vi "Teleop.vi"(10 "Match Info":T1={"Autonomous Elapsed Seconds"=0.0, "TeleOp Elapsed Seconds"=0.0, "Disabled Elapsed Seconds"=0.0, "Visited Autonomous"=FALSE, "Visited TeleOp"=FALSE, "Visited Disabled"=FALSE, "Autonomous Settings"={"Autonomous Style"=enum."Independent", "VI Refnum"=refnum}}, 11 "Call Context":T2) -> ()   [LabVIEW 2013]
doc: "This VI is called for each TeleOp packet received from the DS where the robot is not disabled. It is often used to read from the joysticks and update I/O or to update setpoints for timed control loops. It should complete and return within 20 milliseconds or it may miss DS packets."
uses:
  <vilib>/Rock Robotics/WPI/DriverStation/WPI_DriverStationDerivedRobotMode.ctl
  <vilib>/Rock Robotics/WPI/DriverStation/WPI_DriverStationMatch Info.ctl
  <vilib>/Rock Robotics/WPI/Solenoid/WPI_SolenoidValue.ctl
  <vilib>/Rock Robotics/WPI/Relay/WPI_RelayValue.ctl
  Robot Global Data.vi
  <vilib>/Rock Robotics/WPI/Joystick/WPI_JoystickGetSetRefNum.vi
  <vilib>/Rock Robotics/WPI/RobotDrive/WPI_RobotDriveGetSetRefNum.vi
  <vilib>/Rock Robotics/WPI/RobotDrive/WPI_RobotDriveArcadeDrive_Standard(NoSaturation).vi
  <vilib>/Rock Robotics/WPI/Solenoid/WPI_SolenoidSetEnum.vi
panel:
  out "Numeric 1":dbl(slide) scale=0.0..100.0
  out "Boolean 2":bool
  out "Boolean 1":bool
  # "display DB vars here"
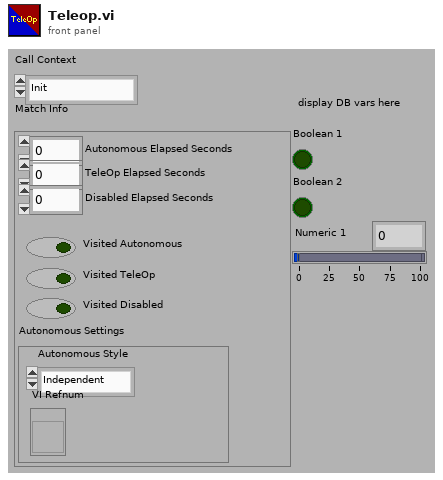
[diagram p1: front panel]
types:
  T1 = typedef "WPI_DriverStationMatch Info.ctl" = cluster{"Autonomous Elapsed Seconds":dbl, "TeleOp Elapsed Seconds":dbl, "Disabled Elapsed Seconds":dbl, "Visited Autonomous":bool, "Visited TeleOp":bool, "Visited Disabled":bool, "Autonomous Settings":cluster{"Autonomous Style":enum16{"Iterative", "Independent"}, "VI Refnum":refnum<vi>}}
  T2 = typedef "WPI_DriverStationDerivedRobotMode.ctl" = enum16{"Init", "Execute", "Stop"}
  T3 = typedef "WPI_JoystickDevRef.ctl" = cluster{"Device":T4}
  T4 = typedef "WPI_JoystickDeviceEnum.ctl" = enum16{"USB 1", "USB 2", "USB 3", "USB 4", "Kinect 1", "Kinect 2"}
  T5 = cluster{"axis 1 (x)":dbl, "axis 2 (y)":dbl, "axis 3 (throttle)":dbl, "axis 4":dbl, "axis 5":dbl, "axis 6":dbl}
  T6 = typedef "WPI_JoystickButtonState.ctl" = cluster{"Button 1":bool, "Button 2":bool, "Button 3":bool, "Button 4":bool, "Button 5":bool, "Button 6":bool, "Button 7":bool, "Button 8":bool, "Button 9":bool, "Button 10":bool, "Button 11":bool, "Button 12":bool}
  T7 = typedef "WPI_PWMDeviceRef.ctl" = cluster{"DeviceStatus":errorcluster, "Digital Module":T8, "PWM Channel":T9}
  T8 = typedef "FPGA_TypedefDigitalModule.ctl" = enum16{"Digital Module 1", "Digital Module 2"}
  T9 = typedef "FPGA_DIOPWMChannel.ctl" = enum8{"PWM 1", "PWM 2", "PWM 3", "PWM 4", "PWM 5", "PWM 6", "PWM 7", "PWM 8", "PWM 9", "PWM 10", "Invalid"}
  T10 = typedef "WPI_DigitalOutputDevRef.ctl" = cluster{"Digital Module":T8, "DIO Channel":T11, "DevStatus":errorcluster}
  T11 = typedef "FPGA_DIOChannel.ctl" = enum8{"DIO 1", "DIO 2", "DIO 3", "DIO 4", "DIO 5", "DIO 6", "DIO 7", "DIO 8", "DIO 9", "DIO 10", "DIO 11", "DIO 12", "DIO 13", "DIO 14", "Invalid"}
  T12 = typedef "WPI_RobotDriveDevRef.ctl" = cluster{"DevStatus":errorcluster, "Motors[]":T13[], "Square Inputs":bool, "Max Output":dbl, "Isochronous":bool}
  T13 = typedef "WPI_MotorControlDeviceRef.ctl" = cluster{"DeviceStatus":errorcluster, "Type":enum16{"PWM", "CAN"}, "PWM":cluster{"Digital Module":T8, "PWM Channel":T9, "DeadBand":T14}, "CAN":cluster{"Device Number":u8, "Control Mode":T15, "Semaphore":T16, "Max Vout":dbl}, "Invert":bool, "TransformRef":T17, "InvTransformRef":T17}
  T14 = typedef "WPI_PWMDeadband.ctl" = cluster{"Name":string, "maxPositivePwm":i32, "minPositivePwm":i32, "centerPwm":i32, "maxNegativePwm":i32, "minNegativePwm":i32, "angularRange":u16}
  T15 = typedef "WPI_CANJaguar_ControlMode.ctl" = enum8{"Percent VBus", "Current", "Speed", "Position", "Voltage"}
  T16 = typedef "Semaphore RefNum" = refnum<k1>
  T17 = typedef "WPI_PWMTransform_ConPane.ctl" = refnum<vi>
  T18 = typedef "WPI_SolenoidValue.ctl" = enum16{"Off", "On", "Forward", "Reverse"}
  T19 = typedef "WPI_RelayValue.ctl" = enum16{"Off", "On", "Forward", "Reverse"}
  T20 = typedef "WPI_RelayDevRef.ctl" = cluster{"DevStatus":errorcluster, "Relay Channel":T21, "Digital Module":T8, "Relay Direction":T22}
  T21 = typedef "FPGA_DIORelayChannel.ctl" = enum8{"Relay 1", "Relay 2", "Relay 3", "Relay 4", "Relay 5", "Relay 6", "Relay 7", "Relay 8", "Invalid"}
  T22 = typedef "WPI_RelayDirection.ctl" = enum16{"Both directions", "Forward only", "Reverse only"}
  T23 = typedef "WPI_SolenoidDevRef.ctl" = cluster{"DevStatus":errorcluster, "Solenoid Module":T24, "Forward Solenoid Channel":T25, "Reverse Solenoid Channel":T25}
  T24 = typedef "FPGA_TypedefSolenoidModule.ctl" = enum16{"Solenoid Module 1", "Solenoid Module 2"}
  T25 = typedef "WPI_SolenoidChannel.ctl" = enum8{"Solenoid 1", "Solenoid 2", "Solenoid 3", "Solenoid 4", "Solenoid 5", "Solenoid 6", "Solenoid 7", "Solenoid 8", "Invalid"}
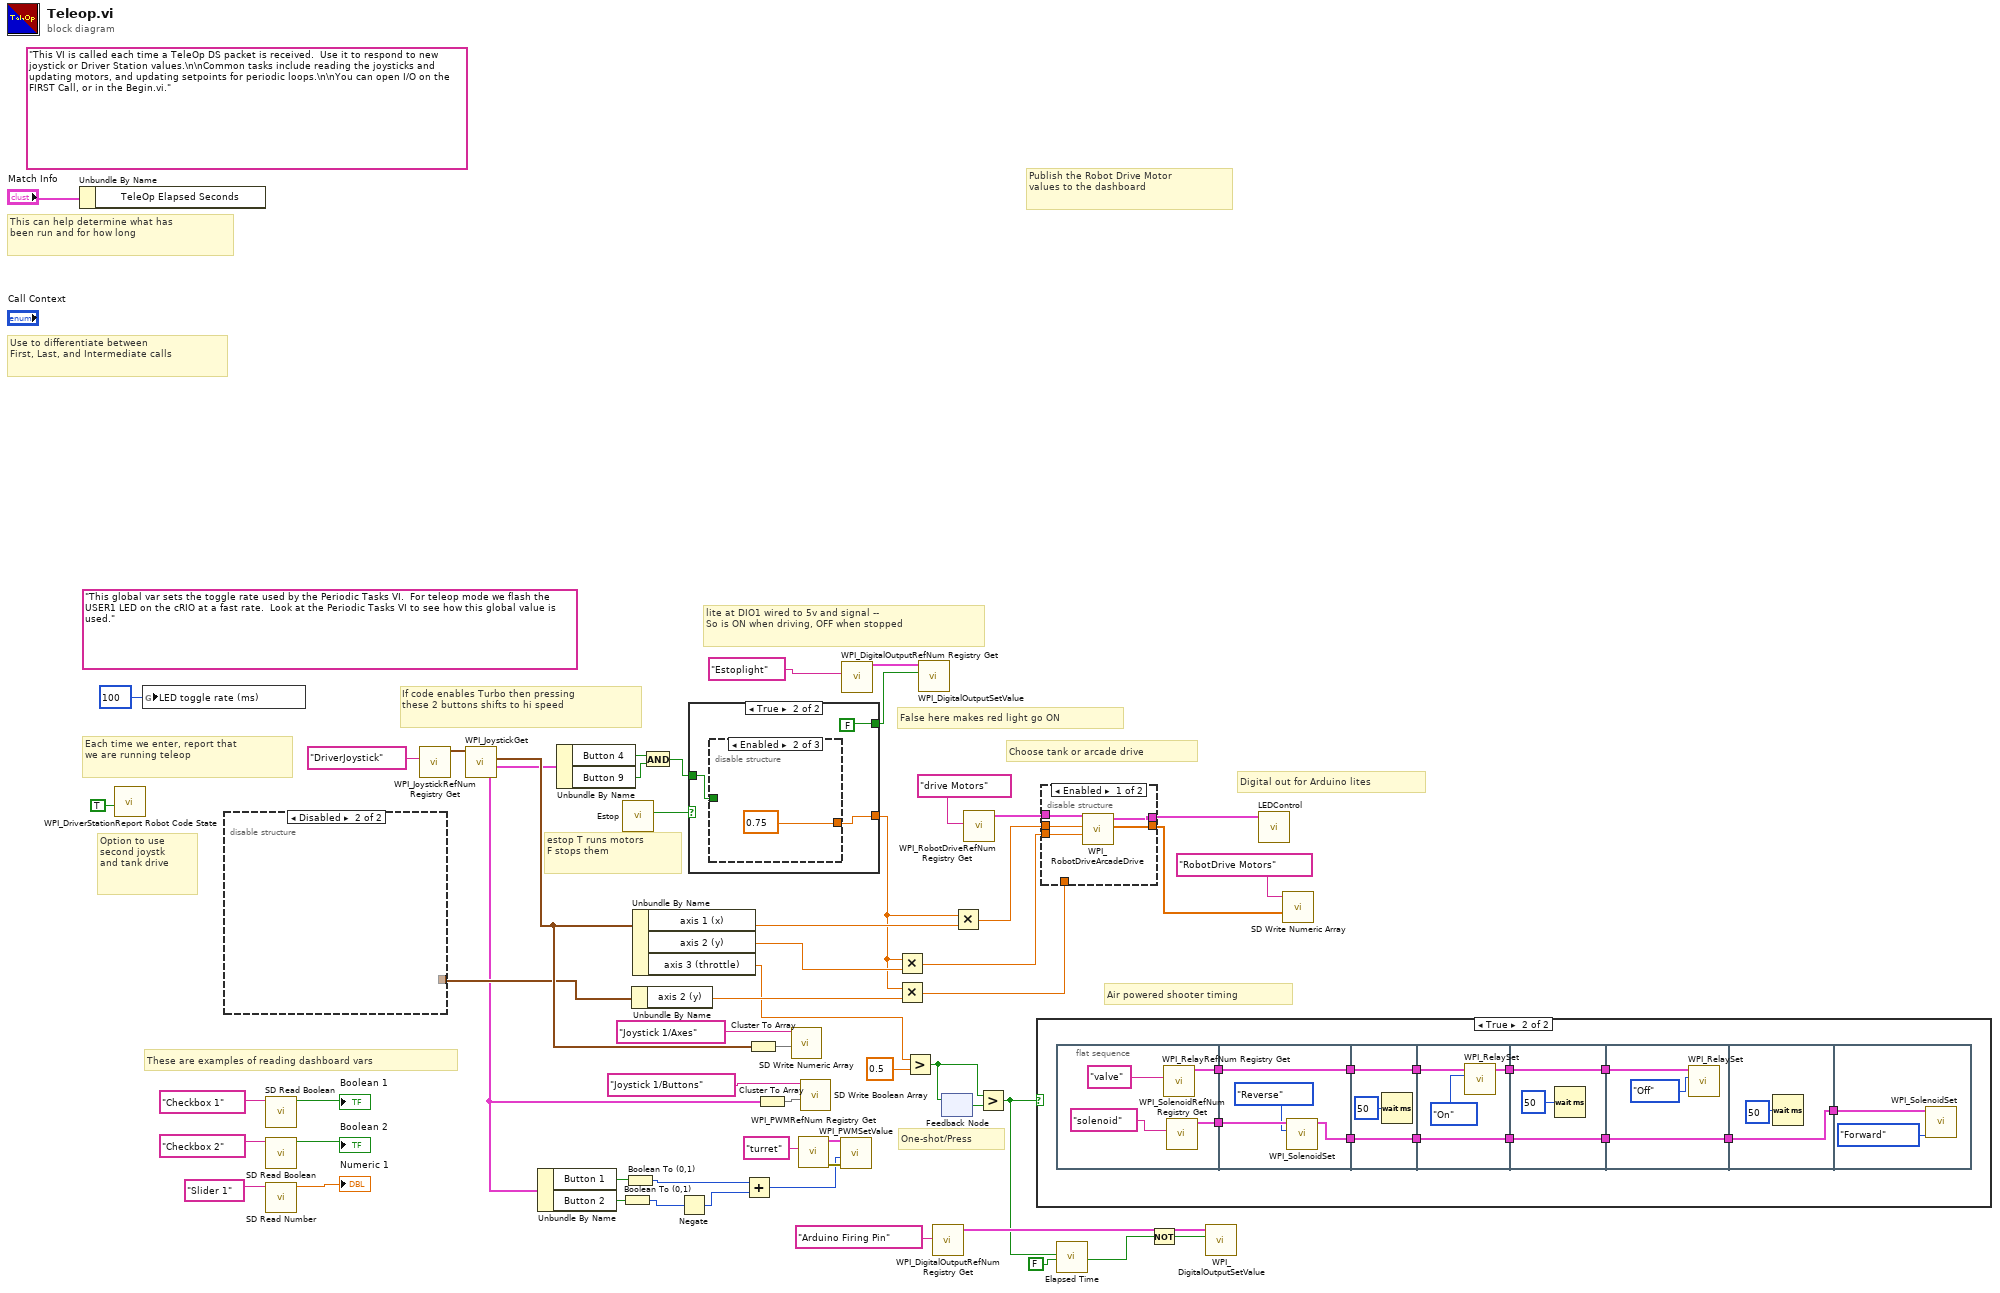
[diagram p0: block diagram]
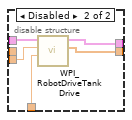
[diagram p3: hidden frame]
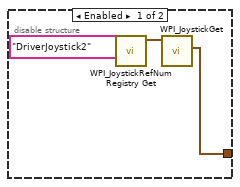
[diagram p4: hidden frame]
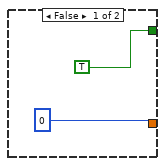
[diagram p5: hidden frame]
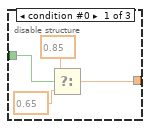
[diagram p6: hidden frame]
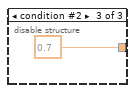
[diagram p7: hidden frame]
diagram:
  (unwired) "This global var sets the toggle rate used by the Periodic Tasks VI.  For teleop mode we flash the USER1 LED on the cRIO at a fast rate.  Look at the Periodic Tasks VI to see how this global value is used."
  (unwired) "This VI is called each time a TeleOp DS packet is received.  Use it to respond to new joystick or Driver Station values.\n\nCommon tasks include reading the joysticks and updating motors, and updating setpoints for periodic loops.\n\nYou can open I/O on the FIRST Call, or in the Begin.vi."
  # "Air powered shooter timing"
  # "False here makes red light go ON"
  # "Option to use\nsecond joystk\nand tank drive"
  # "One-shot/Press"
  # "estop T runs motors\nF stops them"
  # "If code enables Turbo then pressing\nthese 2 buttons shifts to hi speed"
  # "lite at DIO1 wired to 5v and signal --\nSo is ON when driving, OFF when stopped"
  # "Choose tank or arcade drive"
  # "Digital out for Arduino lites"
  # "These are examples of reading dashboard vars"
  # "Publish the Robot Drive Motor\nvalues to the dashboard"
  # "Each time we enter, report that\nwe are running teleop"
  # "Use to differentiate between\nFirst, Last, and Intermediate calls"
  # "This can help determine what has\nbeen run and for how long"
  n1 = Unbundle By Name("Match Info") -> ()  [unwired: 1 out]
  n2 = call <vilib>:"WPI_DriverStationReport Robot Code State.vi"("TeleOp"=TRUE ("Autonomous")) -> ()  [unwired: 10 in, 1 out]
  n3 = global write "Robot Global Data.vi" "LED toggle rate (ms)"(u32 100 ("LED ms toggle rate")) -> ()
  n4 = disable-structure shown="Disabled" {
    disable-tunnel: [w57 _] -> w26
    frame Enabled {
      n5 = call <vilib>:"WPI_JoystickRefNum Registry Get.vi"("refnum name"="DriverJoystick2") -> ("JoystickDevRef"=w58:T3)  [unwired: 9 in, 1 out]
      n6 = call <vilib>:"WPI_JoystickGet.vi"("JoystickDevRef"=w58) -> ("Axes"=w57:T5)  [unwired: 4 in, 2 out]
    }
    frame Disabled {
    }
  }
  n7 = call <vilib>:"SD Read Boolean.vi"("Name"="Checkbox 1" ("refnum name")) -> ("Boolean"=→"Boolean 1":bool)  [unwired: 8 in, 2 out]
  n8 = call <vilib>:"SD Read Boolean.vi"("Name"="Checkbox 2" ("refnum name")) -> ("Boolean"=→"Boolean 2":bool)  [unwired: 8 in, 2 out]
  n9 = call <vilib>:"SD Read Number.vi"("Name"="Slider 1" ("refnum name")) -> ("Numeric"=→"Numeric 1":dbl)  [unwired: 8 in, 2 out]
  n10 = call <vilib>:"WPI_JoystickRefNum Registry Get.vi"("refnum name"="DriverJoystick") -> ("JoystickDevRef"=w44:T3)  [unwired: 9 in, 1 out]
  n11 = call <vilib>:"WPI_JoystickGet.vi"("JoystickDevRef"=w44) -> ("Buttons"=w20:T6, "Axes"=w28:T5)  [unwired: 4 in, 1 out]
  n12 = Unbundle By Name(w20) -> ("Button 1"=w19:bool, "Button 2"=w18:bool)
  n13 = Unbundle By Name(w20) -> ("Button 4"=w42:bool, "Button 9"=w41:bool)
  n14 = Boolean To (0,1)(Boolean=w18) -> (0, 1=w16:i16)
  n15 = call "Estop.vi"() -> ("Estop?"=w43:bool)  [unwired: 11 in]
  n16 = Boolean To (0,1)(Boolean=w19) -> (0, 1=w17:i16)
  n17 = Unbundle By Name(w26) -> ("axis 2 (y)"=w22:dbl)
  n18 = Unbundle By Name(w28) -> ("axis 1 (x)"=w39:dbl, "axis 2 (y)"=w25:dbl, "axis 3 (throttle)"=w10:dbl)
  n19 = And(x=w42, y=w41) -> (x .and. y?=w40:bool)
  n20 = Negate(x=w16) -> (-x=w15:i16)
  n21 = case shown="True" w43 {
    tunnel: w40 -> [_ w64]
    tunnel: [0 w63] -> w23
    tunnel: [TRUE FALSE] -> w35
    frame False {
    }
    frame True {
      n22 = disable-structure shown="Enabled" {
        disable-tunnel: w64 -> [w68 _ _]
        disable-tunnel: [w65 0.75 ("t") 0.7 ("t")] -> w63
        frame condition #0 {
          n23 = Select(t=0.85, s=w68, f=0.65) -> (s? t:f=w65:dbl)
        }
        frame condition #1 (active) {
        }
        frame condition #2 {
        }
      }
    }
  }
  n24 = Add(x=w17, y=w15) -> (x+y=w11:i16)
  n25 = Cluster To Array(cluster=w28) -> (array=w31:dbl[])
  n26 = Cluster To Array(cluster=w20) -> (array=w32:bool[])
  n27 = call <vilib>:"SD Write Numeric Array.vi"("Numeric Array"=w31, "Name"="Joystick 1/Axes") -> ()  [unwired: 8 in, 2 out]
  n28 = call <vilib>:"WPI_PWMRefNum Registry Get.vi"("refnum name"="turret") -> ("error out"=w13:errorcluster, "PWMDeviceRef"=w12:T7)  [unwired: 9 in]
  n29 = call <vilib>:"SD Write Boolean Array.vi"("Boolean Array"=w32, "Name"="Joystick 1/Buttons") -> ()  [unwired: 8 in, 2 out]
  n30 = call <vilib>:"WPI_PWMSetValue.vi"("error in (no error)"=w13, "Value"=w11, "PWMDeviceRef"=w12) -> ()  [unwired: 7 in, 2 out]
  n31 = call <vilib>:"WPI_DigitalOutputRefNum Registry Get.vi"("refnum name"="Estoplight") -> ("DigitalOutputDevRef"=w36:T10)  [unwired: 9 in, 1 out]
  n32 = Multiply(x=w23, y=w25) -> (x*y=w24:dbl)
  n33 = Multiply(x=w23, y=w22) -> (x*y=w21:dbl)
  n34 = Greater?(x=w10, y=0.5) -> (0:w7:bool)
  n35 = call <vilib>:"WPI_DigitalOutputSetValue.vi"("Value"=w35, "DigitalOutputDevRef"=w36) -> ()  [unwired: 8 in, 2 out]
  n36 = call <vilib>:"WPI_DigitalOutputRefNum Registry Get.vi"("refnum name"="Arduino Firing Pin") -> ("DigitalOutputDevRef"=w5:T10)  [unwired: 9 in, 1 out]
  n37 = feedback-in #1(w7) -> ()
  n38 = feedback #1() -> (w8:bool)  [unwired: 1 in]
  n39 = Multiply(x=w23, y=w39) -> (x*y=w38:dbl)
  n40 = call <vilib>:"WPI_RobotDriveRefNum Registry Get.vi"("refnum name"="drive Motors") -> ("RobotDriveDevRef"=w46:T12)  [unwired: 9 in, 1 out]
  n41 = Greater?(x=w7, y=w8) -> (0:w4:bool)
  n42 = case shown="True" w4 {
    frame False {
    }
    frame True {
      n43 = flat-sequence {
        tunnel: [w84] -> w82
        tunnel: [w83] -> w81
        tunnel: w82 -> [w90]
        tunnel: [w88] -> w80
        tunnel: w81 -> [w88]
        tunnel: [w87] -> w72
        tunnel: w80 -> [w93]
        tunnel: [w93] -> w79
        tunnel: [w91] -> w73
        tunnel: w72 -> [w91]
        tunnel: w79 -> [w97]
        tunnel: [w95] -> w78
        tunnel: [w94] -> w74
        tunnel: w73 -> [w94]
        tunnel: w78 -> [w99]
        tunnel: [w99] -> w77
        tunnel: [w98] -> w75
        tunnel: w74 -> [w98]
        tunnel: w77 -> [w102]
        tunnel: [w101] -> w76
        tunnel: w75 -> [w101]
        tunnel: w76 -> [w104]
        tunnel: [w104] -> w71
        tunnel: w71 -> [w106]
        frame #0 {
          n44 = call <vilib>:"WPI_RelayRefNum Registry Get.vi"("refnum name"="valve") -> ("RelayDevRef"=w83:T20)  [unwired: 9 in, 1 out]
          n45 = call <vilib>:"WPI_SolenoidRefNum Registry Get.vi"("refnum name"="solenoid") -> ("SolenoidDevRef"=w84:T23)  [unwired: 9 in, 1 out]
        }
        frame #1 {
          n46 = call-poly <vilib>:"WPI_SolenoidSet.vi"("Value"=WPI_SolenoidValue."Reverse", "SolenoidDevRef"=w90) -> ("SolenoidDevRef"=w87:T23)  [unwired: 8 in, 1 out]
        }
        frame #2 {
          n47 = Wait (ms)(milliseconds to wait=u32 50) -> ()  [unwired: 1 out]
        }
        frame #3 {
          n48 = call <vilib>:"WPI_RelaySet.vi"("RelayValue"=WPI_RelayValue."On", "RelayDevRef"=w97) -> ("RelayDevRef"=w95:T20)  [unwired: 8 in, 1 out]
        }
        frame #4 {
          n49 = Wait (ms)(milliseconds to wait=u32 50) -> ()  [unwired: 1 out]
        }
        frame #5 {
          n50 = call <vilib>:"WPI_RelaySet.vi"("RelayValue"=WPI_RelayValue."Off", "RelayDevRef"=w102) -> ()  [unwired: 8 in, 2 out]
        }
        frame #6 {
          n51 = Wait (ms)(milliseconds to wait=u32 50) -> ()  [unwired: 1 out]
        }
        frame #7 {
          n52 = call-poly <vilib>:"WPI_SolenoidSet.vi"("Value"=WPI_SolenoidValue."Forward", "SolenoidDevRef"=w106) -> ()  [unwired: 8 in, 2 out]
        }
      }
    }
  }
  n53 = disable-structure shown="Enabled" {
    disable-tunnel: w46 -> [w112 w115]
    disable-tunnel: w38 -> [w111 _]
    disable-tunnel: w24 -> [w110 w114]
    disable-tunnel: [w109 w117] -> w29
    disable-tunnel: [w108 w116] -> w27
    disable-tunnel: w21 -> [_ w113]
    frame Enabled {
      n54 = call-poly <vilib>:"WPI_RobotDriveArcadeDrive.vi"("Y axis value"=w110, "X axis value"=w111, "RobotDriveDevRef"=w112) -> ("Motor Values"=w109:dbl[], "RobotDriveDevRef"=w108:T12)  [unwired: 6 in, 1 out]
    }
    frame Disabled {
      n55 = call <vilib>:"WPI_RobotDriveTankDrive.vi"("Right axis value"=w113, "Left axis value"=w114, "RobotDriveDevRef"=w115) -> ("Motor Values"=w117:dbl[], "RobotDriveDevRef"=w116:T12)  [unwired: 6 in, 1 out]
    }
  }
  n56 = call "Elapsed Time"("Reset"=w4, "Auto Reset"=FALSE) -> ("Time has Elapsed"=w3:bool)  [unwired: 10 in, 7 out]
  n57 = Not(x=w3) -> (.not. x?=w2:bool)
  n58 = call <vilib>:"WPI_DigitalOutputSetValue.vi"("Value"=w2, "DigitalOutputDevRef"=w5) -> ()  [unwired: 8 in, 2 out]
  n59 = call "LEDControl.vi"("RobotDriveDevRef 2"=w27) -> ()  [unwired: 11 in]
  n60 = call <vilib>:"SD Write Numeric Array.vi"("Numeric Array"=w29, "Name"="RobotDrive Motors") -> ()  [unwired: 8 in, 2 out]
